vi "serial tcsetattr.vi"(8 "error in (no error)":errorcluster, 10 "data":string, 11 "portHandle in":i32) -> (0 "error out":errorcluster, 1 "return value":i32, 3 "portHandle out":i32)   [LabVIEW 2016]
uses:
  libc.so.6
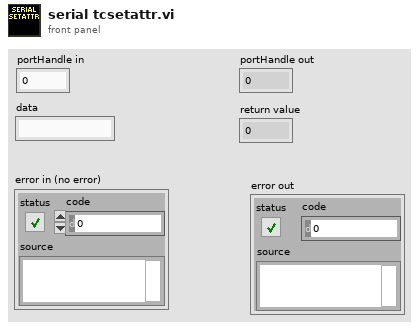
[diagram p1: front panel]
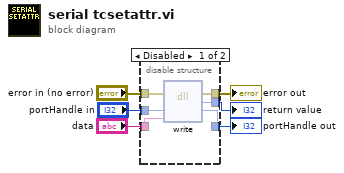
[diagram p0: block diagram]
diagram:
  n1 = disable-structure shown="Disabled" {
    disable-tunnel: [w12 w13] -> w6
    disable-tunnel: "error in (no error)" -> [w11 w13]
    disable-tunnel: "portHandle in" -> [w10 _]
    disable-tunnel: "data" -> [w9 _]
    disable-tunnel: [w8 _] -> w2
    disable-tunnel: [w7 _] -> w1
    frame Disabled {
      n2 = dll-call lib="libc.so.6" fn="write"(error in=w11, "portHandle"=w10, "data"=w9) -> (error out=w12:errorcluster, "return type"=w7:i32, "portHandle"=w8:i32)  [unwired: 3 in, 1 out]
    }
    frame Enabled {
    }
  }
  "error out" <- w6
  "portHandle out" <- w2
  "return value" <- w1
